vi "Test_Stop Service.vi"() -> ()   [LabVIEW 2020]
uses:
  Measurement_client/RPC Messages/ni_servicemanagement_v1_StopServiceRequest.ctl
  Measurement_client/Measurement_client.lvlib
panel:
  in  "address":string
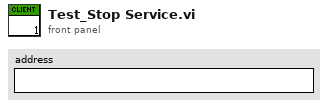
[diagram p1: front panel]
types:
  T1 = typedef "Measurement_client.lvlib/ni_servicemanagement_v1_StopServiceRequest.ctl" = cluster{"void":string}
  T2 = typedef "gprc-lvsupport-release.lvlib/grpcId.ctl" = u64
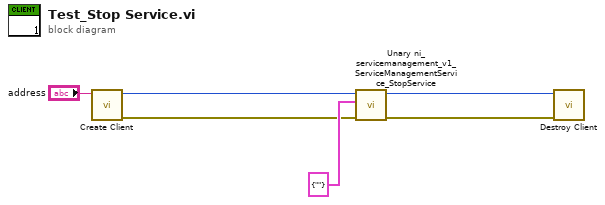
[diagram p0: block diagram]
diagram:
  n1 = call "Create Client.vi"("address"="address") -> ("error out"=w2:errorcluster, "gRPC ID Out"=w6:T2)  [unwired: 9 in]
  n2 = call "Unary ni_servicemanagement_v1_ServiceManagementService_StopService.vi"("error in"=w2, "Request Data"=T1 {"void"=""}, "gRPC ID"=w6) -> ("error out"=w3:errorcluster, "gRPC ID out"=w5:T2)  [unwired: 6 in, 1 out]
  n3 = call "Destroy Client.vi"("error in"=w3, "gRPC ID"=w5) -> ()  [unwired: 9 in, 1 out]
